vi "Prompt for Step.vi"(8 "error in (no error)":errorcluster, 9 "Index":i32=-1, 11 "Steps":refnum<class "Step.lvclass">[](array[class])) -> (0 "error out":errorcluster, 1 "OK?":bool, 3 "Step":refnum<class "Step.lvclass">)   [LabVIEW 2020, in "MacroAssert.lvlib"]
doc: "Prompts to enter a new step in the profile."
uses:
  MacroAssert.lvlib
  Classes/Step/Step.lvclass
  Classes/Macro/Macro.lvclass
  CTLs/Prompt for Step State Data.ctl
  FaKI State Machine/FaKI State Machine.lvlib
  CTLs/Step Type V3.ctl
panel:
  in  "Save Default":bool
  in  "Step Notes":string
  out "Step Type Description":string
  in  "Repeat":i32 min=0
  in  "Delay":i32=100 min=0
  in  "Step Type":T1
  in  "Cancel":bool
  in  "OK":bool
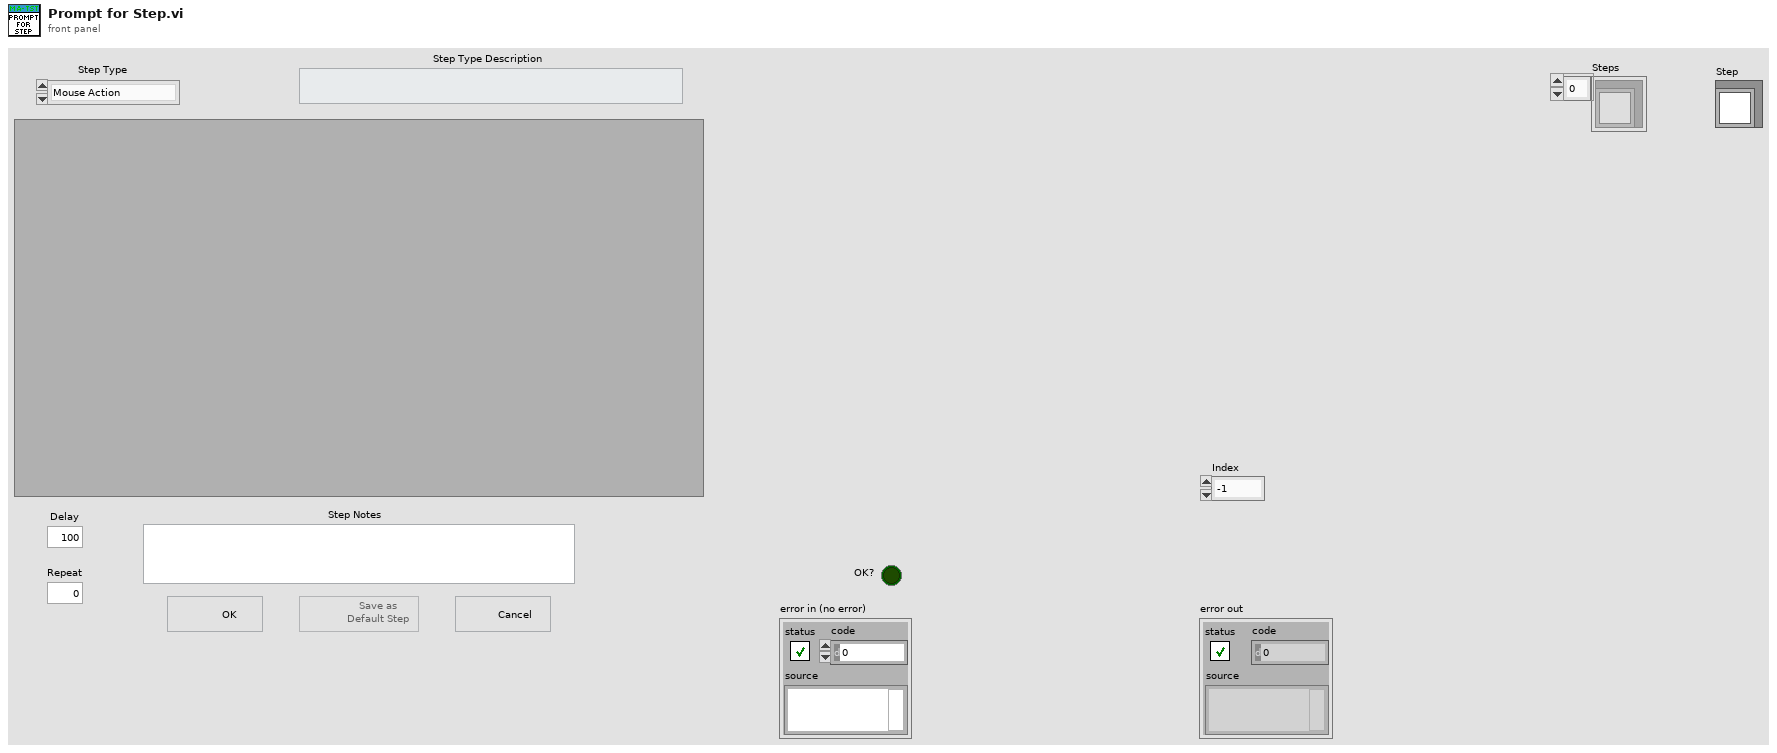
[diagram p1: front panel]
types:
  T1 = typedef "MacroAssert.lvlib/Step Type V3.ctl" = enum16{"Mouse Action", "Keyboard Action", "Window Action", "Timing Action", "Boolean Assertion", "Numeric Assertion", "String Assertion", "Image Assertion"}
  T2 = typedef "MacroAssert.lvlib/Prompt for Step State Data.ctl" = cluster{"Core":cluster{"Current VI Reference":refnum<vi>, "Close Panel on Exit?":bool}, "Mouse Ref":refnum<k1>, "Step":refnum<class "Step.lvclass">, "OK?":bool}
  T3 = enum32{"Invalid", "Standard", "Closed", "Hidden", "Minimized", "Maximized"}
  T4 = enum32{"invalid app kind", "Development System", "Run Time System", "Student Edition", "Embedded LabVIEW", "Evaluation", "Custom"}
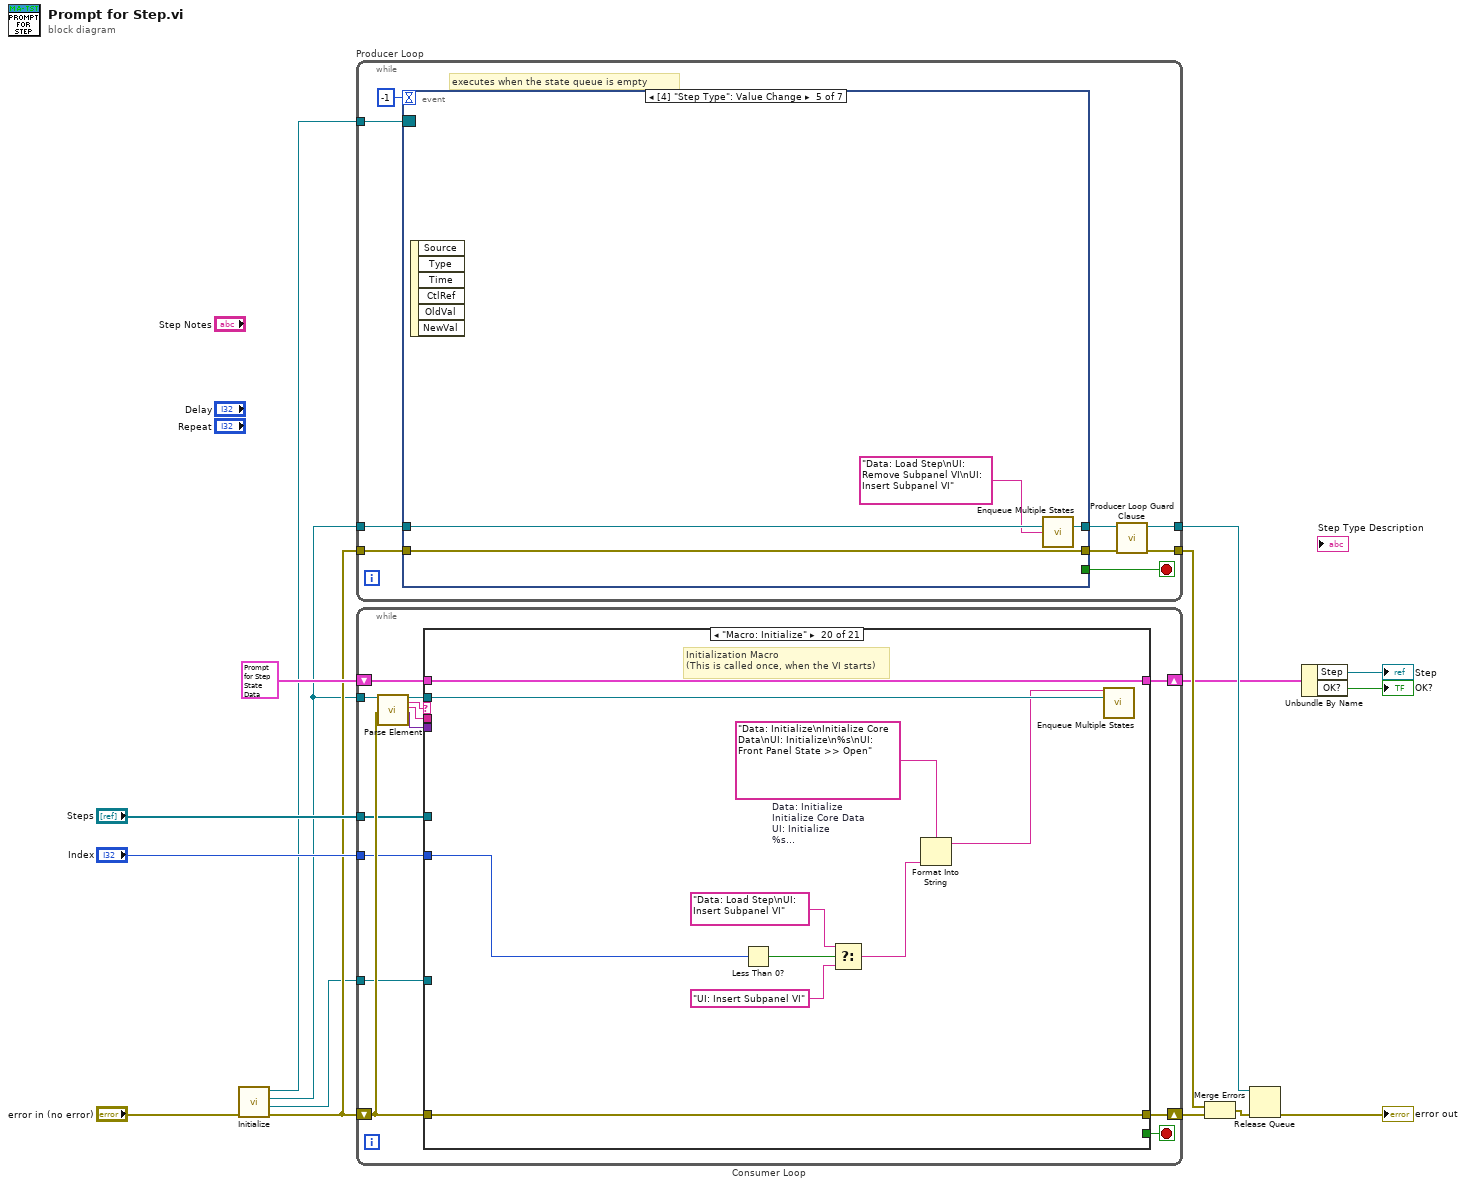
[diagram p0: block diagram]
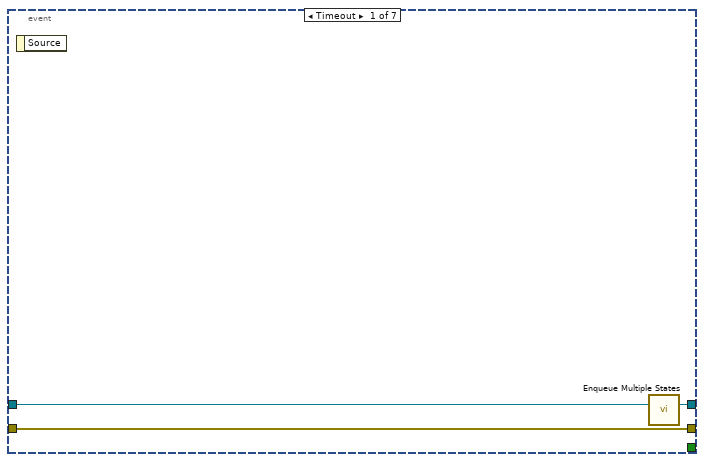
[diagram p2: hidden frame]
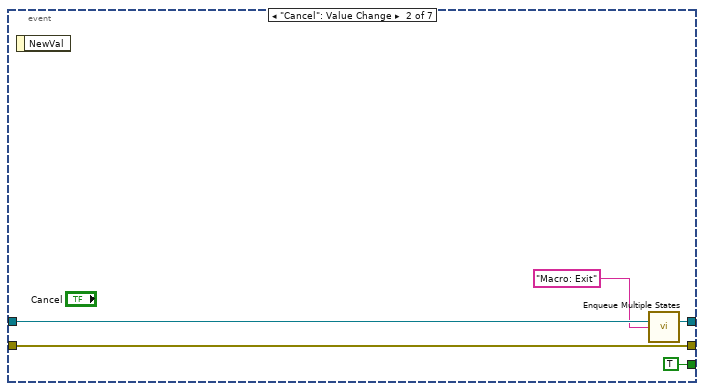
[diagram p3: hidden frame]
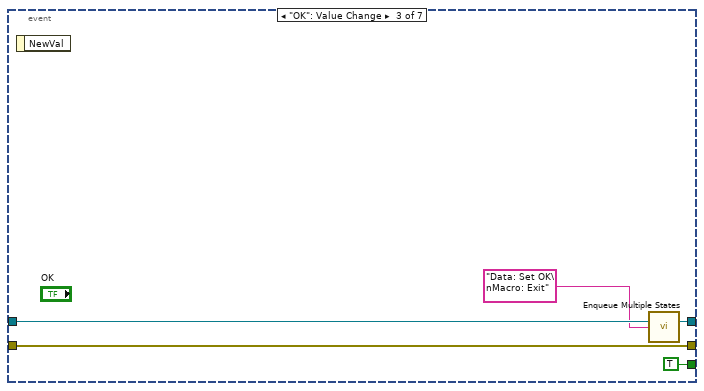
[diagram p4: hidden frame]
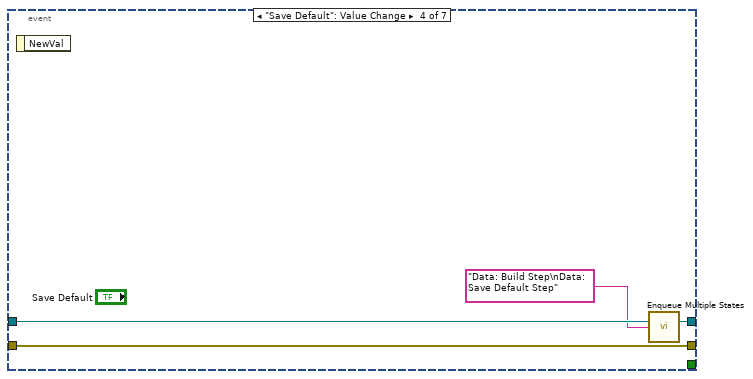
[diagram p5: hidden frame]
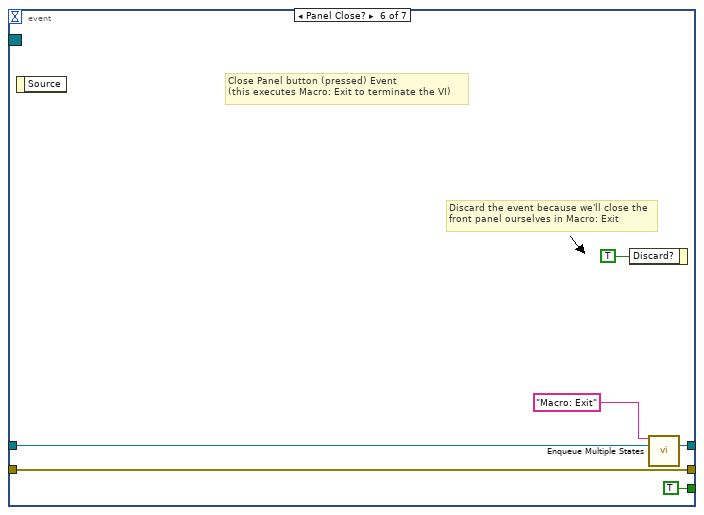
[diagram p6: hidden frame]
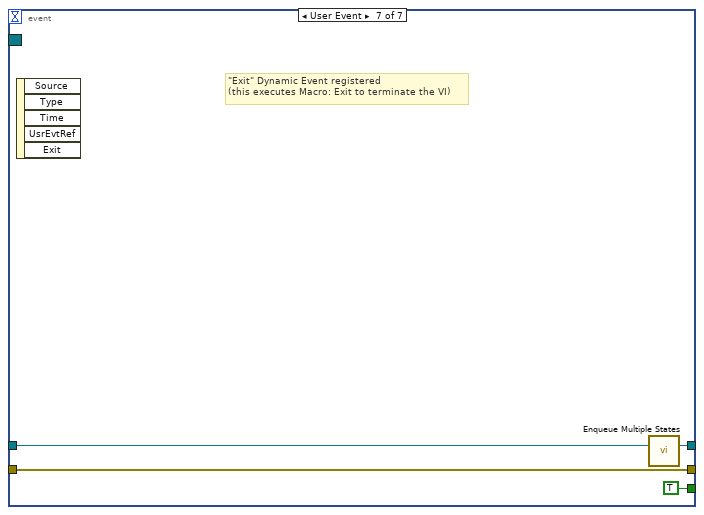
[diagram p7: hidden frame]
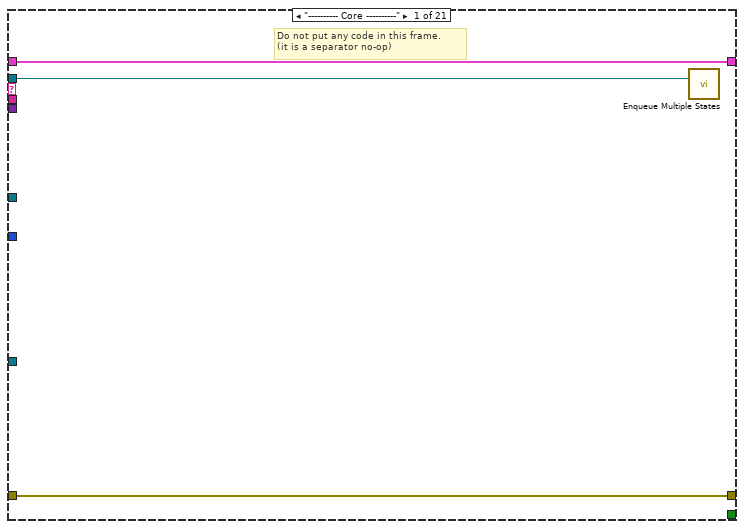
[diagram p8: hidden frame]
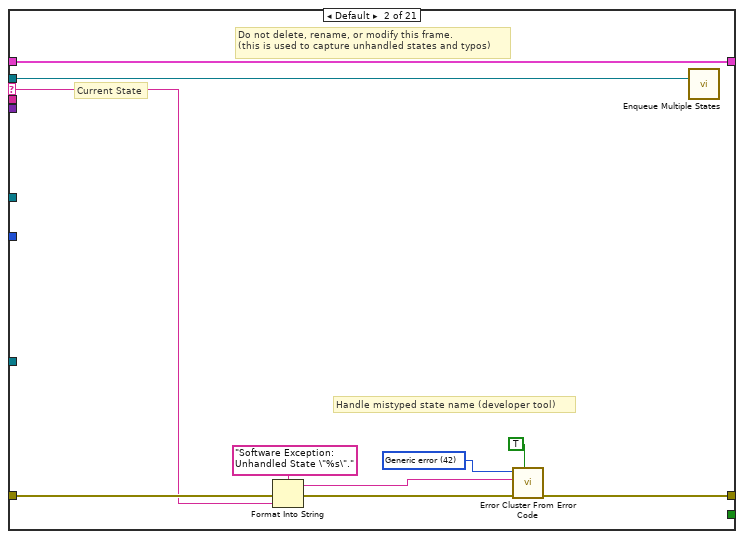
[diagram p9: hidden frame]
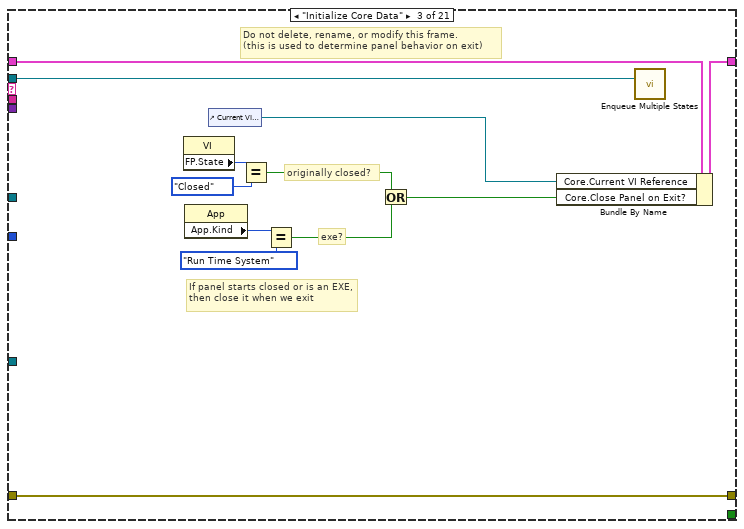
[diagram p10: hidden frame]
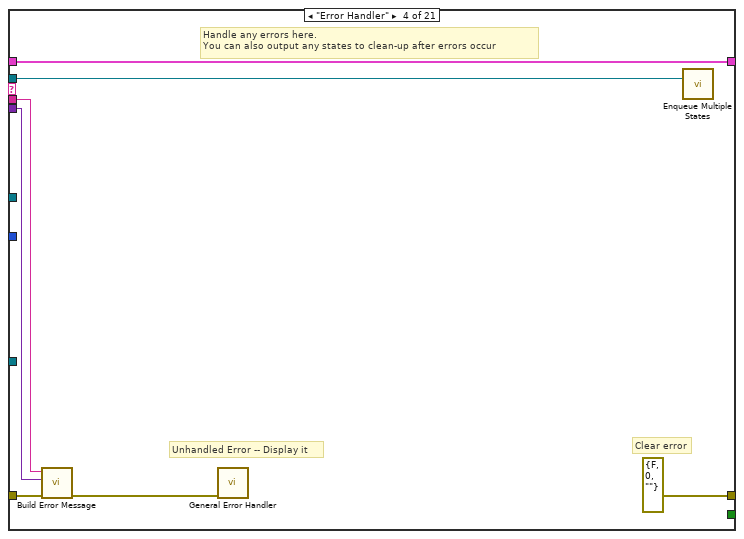
[diagram p11: hidden frame]
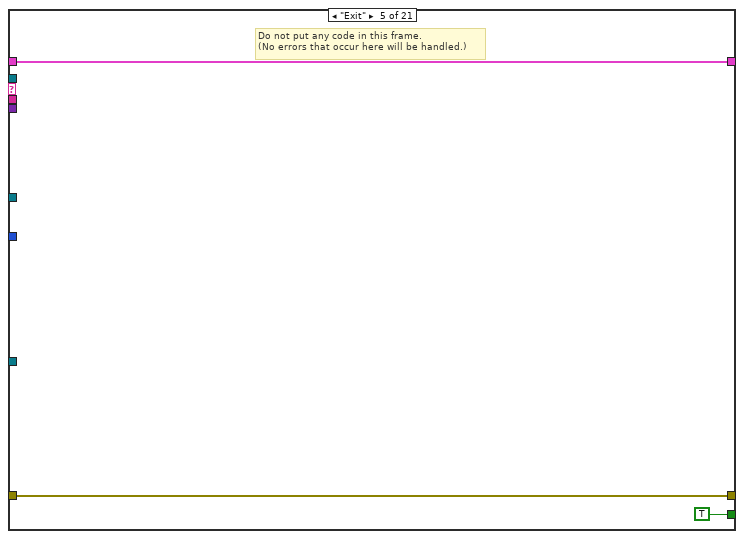
[diagram p12: hidden frame]
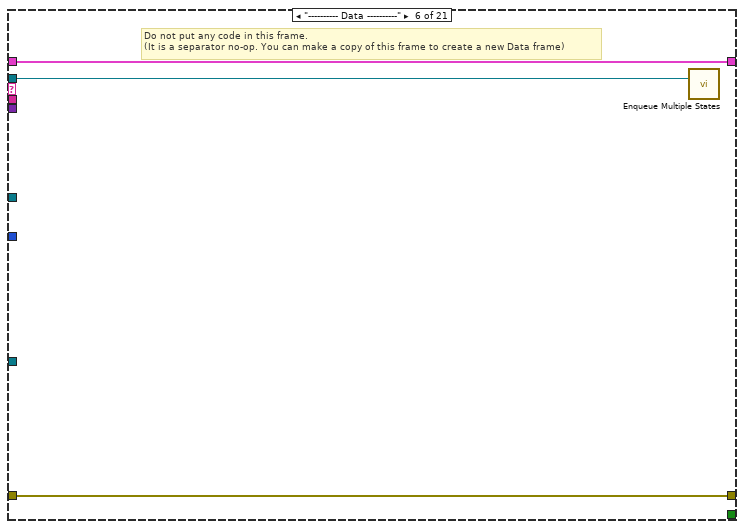
[diagram p13: hidden frame]
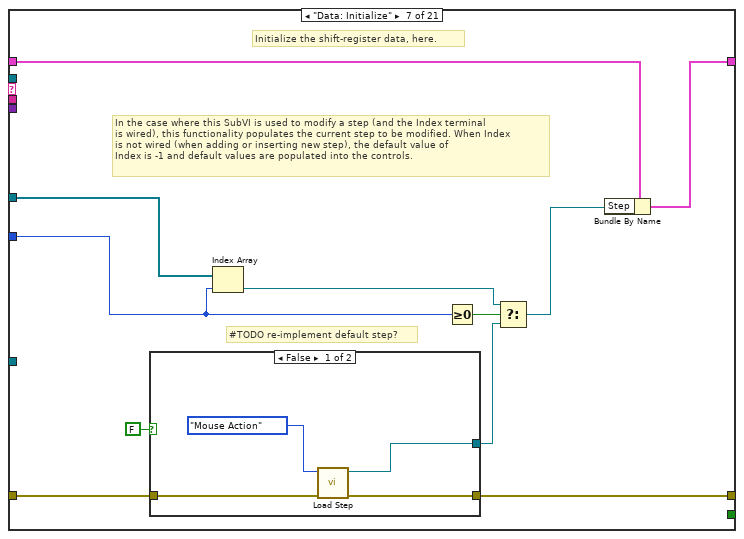
[diagram p14: hidden frame]
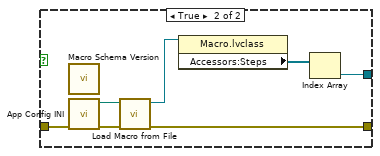
[diagram p15: hidden frame]
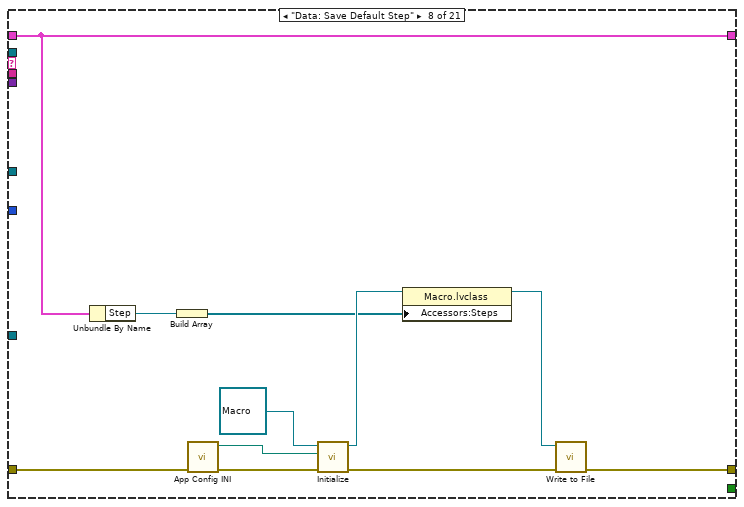
[diagram p16: hidden frame]
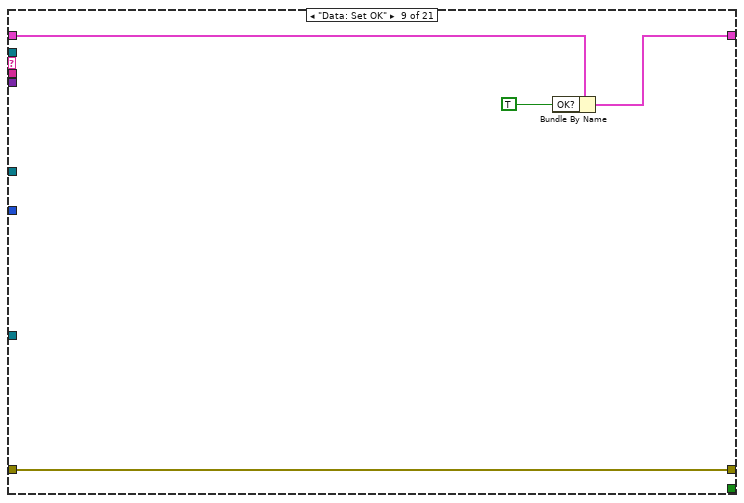
[diagram p17: hidden frame]
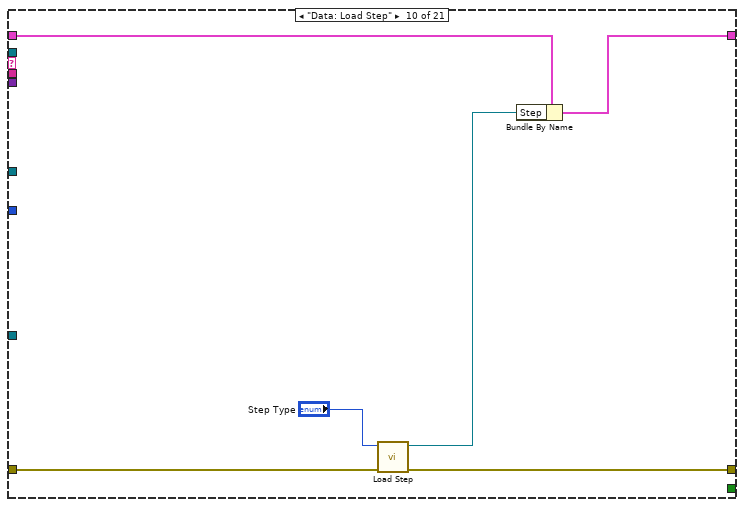
[diagram p18: hidden frame]
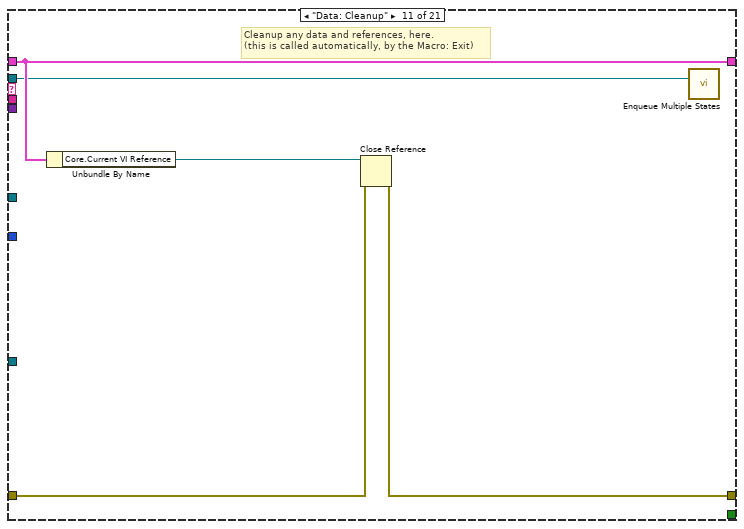
[diagram p19: hidden frame]
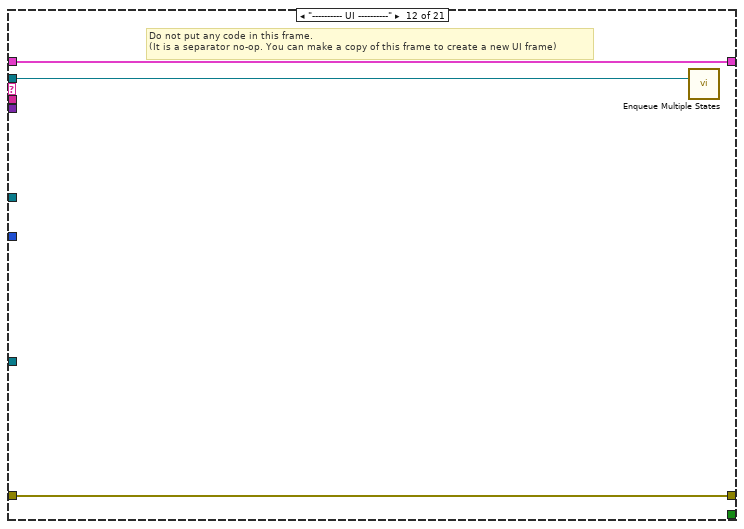
[diagram p20: hidden frame]
diagram:
  n1 = call "Initialize.vi"("error in (no error)"="error in (no error)") -> ("error out"=w6:errorcluster, "Exit Event"=w2:refnum<user-event>, "Queue"=w5:refnum<queue>, "Event Registration Refnum"=w4:refnum<event-registration>)  [unwired: 7 in]
  n2 = while "Producer Loop" {
    tunnel: w4 -> [w17]
    tunnel: w5 -> [w21]
    tunnel: [w18] -> w12
    tunnel: w6 -> [w25]
    tunnel: [w23] -> w15
    stop <- w20 stop-if-true
    # "executes when the state queue is empty"
    n3 = event shown="[4] \"Step Type\": Value Change" {
      selector: w17 -> [_ _ _ _ _ _ _]
      dyn-events: _ -> [_ _ _ _ _ _ _]
      timeout: -1 ("Timeout") -> [_ _ _ _ _ _ _]
      tunnel: [w28 w33 w38 w42 w46 w52 w56] -> w24
      tunnel: w25 -> [w28 w33 w38 w42 w46 w52 w56]
      tunnel: w21 -> [w26 w32 w37 w41 w45 w49 w55]
      tunnel: [w27 w31 w36 w40 w44 w48 w54] -> w19
      tunnel: [_ TRUE TRUE _ _ TRUE TRUE] -> w20
      event Timeout {
        n4 = event-data() -> ()  [unwired: 1 in, 1 out]
        n5 = call "Enqueue Multiple States.vi"("queue in"=w26) -> ("queue out"=w27:refnum<queue>)  [unwired: 14 in]
      }
      event "Cancel": Value Change {
        n6 = event-data() -> ()  [unwired: 1 in, 1 out]
        n7 = call "Enqueue Multiple States.vi"("queue in"=w32, "State(s) at Back"="Macro: Exit") -> ("queue out"=w31:refnum<queue>)  [unwired: 13 in]
      }
      event "OK": Value Change {
        n8 = event-data() -> ()  [unwired: 1 in, 1 out]
        n9 = call "Enqueue Multiple States.vi"("queue in"=w37, "State(s) at Back"="Data: Set OK\nMacro: Exit") -> ("queue out"=w36:refnum<queue>)  [unwired: 13 in]
      }
      event "Save Default": Value Change {
        n10 = event-data() -> ()  [unwired: 1 in, 1 out]
        n11 = call "Enqueue Multiple States.vi"("queue in"=w41, "State(s) at Back"="Data: Build Step\nData: Save Default Step") -> ("queue out"=w40:refnum<queue>)  [unwired: 13 in]
      }
      event Value Change {
        n12 = event-data() -> ()  [unwired: 1 in, 6 out]
        n13 = call "Enqueue Multiple States.vi"("queue in"=w45, "State(s) at Back"="Data: Load Step\nUI: Remove Subpanel VI\nUI: Insert Subpanel VI") -> ("queue out"=w44:refnum<queue>)  [unwired: 13 in]
      }
      event Panel Close? {
        # "Discard the event because we'll close the front panel ourselves in Macro: Exit"
        # "Close Panel button (pressed) Event\n(this executes Macro: Exit to terminate the VI)"
        n14 = event-data() -> ()  [unwired: 1 in, 1 out]
        n15 = event-data("Discard?"=TRUE) -> ()  [unwired: 1 in, 1 out]
        n16 = call "Enqueue Multiple States.vi"("State(s) at Front"="Macro: Exit", "queue in"=w49) -> ("queue out"=w48:refnum<queue>)  [unwired: 13 in]
      }
      event User Event {
        # "\"Exit\" Dynamic Event registered\n(this executes Macro: Exit to terminate the VI)"
        n17 = event-data() -> ()  [unwired: 1 in, 5 out]
        n18 = call "Enqueue Multiple States.vi"("queue in"=w55) -> ("queue out"=w54:refnum<queue>)  [unwired: 14 in]
      }
    }
    n19 = call "Producer Loop Guard Clause.vi"("error in (no error)"=w24, "queue in"=w19) -> ("error out"=w23:errorcluster, "queue out"=w18:refnum<queue>)  [unwired: 8 in]
  }
  n20 = while "Consumer Loop" {
    shift-right: [w66] -> w8
    shift-left: T2 {"Core"={"Current VI Reference"=refnum, "Close Panel on Exit?"=FALSE}, "Mouse Ref"=refnum, "Step"=refnum, "OK?"=FALSE} ("Prompt for Step State Data") -> [w57]
    shift-right: [w69] -> w16
    shift-left: w6 -> [w68]
    tunnel: w5 -> [w65]
    tunnel: w2 -> [w60]
    tunnel: "Steps" -> [w59]
    tunnel: "Index" -> [w58]
    stop <- w67 stop-if-true
    n21 = call "Parse Element.vi"("queue in"=w65, "error in (no error)"=w68) -> ("queue out"=w64:refnum<queue>, "State"=w63:string, "Arg"=w62:string, "Data"=w61:variant)  [unwired: 14 in]
    n22 = case shown="\"Macro: Initialize\"" w63 {
      selector: w63 -> [_ w74 _ _ _ _ _ _ _ _ _ _ _ _ _ _ _ _ _ _ _]
      tunnel: w64 -> [w70 w73 w83 w97 _ w105 _ _ _ _ w152 w156 w161 w164 w165 w174 _ _ w258 w269 w279]
      tunnel: w62 -> [_ _ _ w95 _ _ _ _ _ _ _ _ _ _ w166 w175 _ _ _ _ _]
      tunnel: w57 -> [w71 w76 w89 w98 w103 w106 w117 w139 w144 w150 w153 w157 w160 w163 w167 w177 w246 w257 w259 w268 w283]
      tunnel: [w72 w81 w94 errorcluster {"status"=FALSE, "code"=0, "source"=""} ("error out") w104 w107 w110 w132 w142 w146 w151 w158 w159 w162 w168 w178 w248 w255 w260 w270 w272] -> w69
      tunnel: w68 -> [w72 w80 w94 w100 w104 w107 w118 w140 w142 w147 w155 w158 w159 w162 w169 w179 w247 w256 w260 w270 w273]
      tunnel: [_ _ _ _ TRUE _ _ _ _ _ _ _ _ _ _ _ _ _ _ _ _] -> w67
      tunnel: [w71 w76 w93 w98 w103 w106 w116 w139 w143 w149 w153 w157 w160 w163 w167 w177 w245 w257 w259 w268 w283] -> w66
      tunnel: w61 -> [_ _ _ w96 _ _ _ _ _ _ _ _ _ _ _ _ _ _ _ _ _]
      tunnel: w60 -> [_ _ _ _ _ _ _ _ _ _ _ _ _ _ _ _ _ _ _ _ w274]
      tunnel: w59 -> [_ _ _ _ _ _ w113 _ _ _ _ _ _ _ _ _ _ _ _ _ _]
      tunnel: w58 -> [_ _ _ _ _ _ w112 _ _ _ _ _ _ _ _ _ _ _ _ w267 _]
      frame "---------- Core ----------" {
        # "Do not put any code in this frame.\n(it is a separator no-op)"
        n23 = call "Enqueue Multiple States.vi"("queue in"=w70) -> ()  [unwired: 14 in, 1 out]
      }
      frame Default {
        w78 = 42 items=["No error", "Argument error", "Memory is full", "Out of zone", "End of file", "File already open", "Generic file I/O error", "File not found", "File permission error", "Disk is full", "Duplicate path", "Too many files open", "System feature not enabled", "Resource file not found", "Cannot add resource", "Resource not found", "Image not found", "Image memory error", "Pen does not exist", "Config type invalid", "Config token not found", "Config parse error", "Config memory error", "Bad external code format", "Bad external code offset", "External code not present", "Null window", "Destroy window error", "Null menu", "Print aborted", "Bad print record", "Print driver error", "Windows error during printing", "Memory error during printing", "Print dialog error", "Generic print error", "Invalid device refnum", "Device not found", "Device parameter error", "Device unit error", "Cannot open device", "Device call aborted", "Generic error", "Cancelled by user", "Object ID too low", "Object ID too high", "Object not in heap", "Unknown heap", "Unknown object (invalid DefProc)", "Unknown object (DefProc not in table)", "Message out of range", "Invalid (null) method", "Unknown message", "Manager call not supported", "Bad address", "Network operation in progress", "Network operation timed out", "Connection is busy", "Network attribute not supported", "Network error", "Address in use", "System out of memory", "Connection aborted", "Connection refused", "Not connected", "Already connected", "Connection closed", "Initialization error (interapplication manager)", "Bad occurrence", "Wait on unbound occurrence handler", "Occurrence queue overflow", "Datalog type conflict", "Unused", "Unrecognized type (interapplication manager)", "Memory corrupt", "Failed to make temporary DLL", "Old CIN version", "Drag socket not found", "Failed to load drop-object", "Failed to register OLE object", "Failed to release OLE object", "Format specifier type mismatch", "Unknown format specifier", "Too few format specifiers", "Too many format specifiers", "Scan failed", "Newer CIN version", "Error converting to variant", "Runtime menu error", "Password tampered", "Variant attribute not found", "Incompatible variant data type", "Event data is not available", "Event Store is not present", "Occurrence is not found", "Event Queue is not created", "Event info is not available", "Refnum passed is NULL", "Error retrieving Class GUID", "Error retrieving CoClass GUID", "Error retrieving TypeLib GUID.", "Bad built application magic bytes.", "Specific driver is different from the specific driver associated with the Logical Name.", "There is no session opened to the class driver.", "Max Error", "MAX - Error with config objects", "MAX - Error loading configuration", "MAX - Group not supported"]
        # "Current State"
        # "Do not delete, rename, or modify this frame.\n(this is used to capture unhandled states and typos)"
        # "Handle mistyped state name (developer tool)"
        n24 = Format Into String(format string="Software Exception: Unhandled State \"%s\"." ("message"), error in=w80, w74) -> (resulting string=w77:string, error out=w82:errorcluster)  [unwired: 1 in]
        n25 = call <vilib>:"Error Cluster From Error Code.vi"("show call chain? (False)"=TRUE, "error in (no error)"=w82, "error message (\"\")"=w77, "error code (0)"=w78) -> ("error out"=w81:errorcluster)  [unwired: 5 in]
        n26 = call "Enqueue Multiple States.vi"("queue in"=w73) -> ()  [unwired: 14 in, 1 out]
      }
      frame "Initialize Core Data" {
        # "Do not delete, rename, or modify this frame.\n(this is used to determine panel behavior on exit)"
        # "originally closed?"
        # "exe?"
        # "If panel starts closed or is an EXE, then close it when we exit"
        n27 = property class="VI"() -> ("FP.State"=w86:T3)  [unwired: 2 in, 2 out]
        n28 = property class="App"() -> ("App.Kind"=w92:T4)  [unwired: 2 in, 2 out]
        n29 = control-ref of="Current VI Reference"() -> (w87:refnum<vi>)
        n30 = Equal?(x=w86, y=T3."Closed" ("Front Panel Window:State")) -> (x = y?=w84:bool)
        n31 = Equal?(x=w92, y=T4."Run Time System" ("Application:Kind")) -> (x = y?=w90:bool)
        n32 = Or(x=w84, y=w90) -> (x .or. y?=w88:bool)
        n33 = Bundle By Name(cluster=w89, "Core.Current VI Reference"=w87, "Core.Close Panel on Exit?"=w88) -> (w93:T2)
        n34 = call "Enqueue Multiple States.vi"("queue in"=w83) -> ()  [unwired: 14 in, 1 out]
      }
      frame "Error Handler" {
        # "Unhandled Error -- Display it"
        # "Handle any errors here.\nYou can also output any states to clean-up after errors occur"
        # "Clear error"
        n35 = call "Build Error Message.vi"("error in (no error)"=w100, "Data"=w96, "Arg"=w95) -> ("error out"=w99:errorcluster)  [unwired: 8 in]
        n36 = call <vilib>:"General Error Handler.vi"("error in (no error)"=w99) -> ()  [unwired: 10 in, 5 out]
        n37 = call "Enqueue Multiple States.vi"("queue in"=w97) -> ()  [unwired: 14 in, 1 out]
      }
      frame "Exit" {
        # "Do not put any code in this frame.\n(No errors that occur here will be handled.)"
      }
      frame "---------- Data ----------" {
        # "Do not put any code in this frame.\n(It is a separator no-op. You can make a copy of this frame to create a new Data frame)"
        n38 = call "Enqueue Multiple States.vi"("queue in"=w105) -> ()  [unwired: 14 in, 1 out]
      }
      frame "Data: Initialize" {
        # "#TODO re-implement default step?"
        # "In the case where this SubVI is used to modify a step (and the Index terminal\nis wired), this functionality populates the current step to be modified. When Index\nis not wired (when adding or inserting new step), the default value of\nIndex is -1 and default values are populated into the controls."
        # "Initialize the shift-register data, here."
        n39 = case shown="False" FALSE {
          tunnel: w118 -> [w122 w129]
          tunnel: [w121 w126] -> w110
          tunnel: [w120 w125] -> w109
          frame False {
            n40 = call "Load Step.vi"("error in (no error)"=w122, "Step Type"=Step_Type_V3."Mouse Action") -> ("error out"=w121:errorcluster, "Step"=w120:refnum<class "Step.lvclass">)  [unwired: 8 in]
          }
          frame True {
            n41 = call "Macro Schema Version.vi"() -> ()  [unwired: 10 in, 2 out]
            n42 = call "App Config INI.vi"("error in (no error)"=w129) -> ("error out"=w128:errorcluster, "App Config"=w127:path)  [unwired: 9 in]
            n43 = call "Load Macro from File.vi"("error in (no error)"=w128, "Path"=w127) -> ("error out"=w126:errorcluster, "Macro"=w124:refnum<class "Macro.lvclass">)  [unwired: 8 in]
            n44 = property class="Macro.lvclass"(reference=w124) -> ("Accessors:Steps"=w123:refnum<class "Step.lvclass">[])  [unwired: 1 in, 2 out]
            n45 = Index Array(array=w123) -> (element=w125:refnum<class "Step.lvclass">)  [unwired: 1 in]
          }
        }
        n46 = Index Array(array=w113, index=w112) -> (element=w115:refnum<class "Step.lvclass">)
        n47 = Greater Or Equal To 0?(x=w112) -> (x >= 0?=w114:bool)
        n48 = Select(t=w115, s=w114, f=w109) -> (s? t:f=w111:refnum<class "Step.lvclass">)
        n49 = Bundle By Name(cluster=w117, "Step"=w111) -> (w116:T2)
      }
      frame "Data: Save Default Step" {
        n50 = Unbundle By Name(w139) -> ("Step"=w138:refnum<class "Step.lvclass">)
        n51 = Build Array(w138) -> (w130:refnum<class "Step.lvclass">[])
        n52 = call "App Config INI.vi"("error in (no error)"=w140) -> ("error out"=w137:errorcluster, "App Config"=w136:path)  [unwired: 9 in]
        n53 = call-dynamic "Initialize.vi"("error in (no error)"=w137, "Path"=w136, "Macro in"=refnum<class "Macro.lvclass"> refnum) -> ("error out"=w134:errorcluster, "Macro out"=w133:refnum<class "Macro.lvclass">)  [unwired: 7 in]
        n54 = property class="Macro.lvclass"(reference=w133, "Accessors:Steps"=w130) -> (reference out=w131:refnum<class "Macro.lvclass">)  [unwired: 1 in, 1 out]
        n55 = call-dynamic "Write to File.vi"("error in (no error)"=w134, "Macro in"=w131) -> ("error out"=w132:errorcluster)  [unwired: 8 in, 1 out]
      }
      frame "Data: Set OK" {
        n56 = Bundle By Name(cluster=w144, "OK?"=TRUE) -> (w143:T2)
      }
      frame "Data: Load Step" {
        n57 = call "Load Step.vi"("error in (no error)"=w147, "Step Type"="Step Type") -> ("error out"=w146:errorcluster, "Step"=w145:refnum<class "Step.lvclass">)  [unwired: 8 in]
        n58 = Bundle By Name(cluster=w150, "Step"=w145) -> (w149:T2)
      }
      frame "Data: Cleanup" {
        # "Cleanup any data and references, here.\n(this is called automatically, by the Macro: Exit)"
        n59 = Unbundle By Name(w153) -> ("Core.Current VI Reference"=w154:refnum<vi>)
        n60 = Close Reference(reference=w154, error in (no error)=w155) -> (error out=w151:errorcluster)
        n61 = call "Enqueue Multiple States.vi"("queue in"=w152) -> ()  [unwired: 14 in, 1 out]
      }
      frame "---------- UI ----------" {
        # "Do not put any code in this frame.\n(It is a separator no-op. You can make a copy of this frame to create a new UI frame)"
        n62 = call "Enqueue Multiple States.vi"("queue in"=w156) -> ()  [unwired: 14 in, 1 out]
      }
      frame "UI: Initialize" {
        # "Initialize the User Interface, here.\n(this is called automatically, by the Macro: Init)"
        n63 = call "Enqueue Multiple States.vi"("queue in"=w161) -> ()  [unwired: 14 in, 1 out]
      }
      frame "UI: Uninitialize" {
        # "Uninitialize the User Interface, here.\n(this is called automatically, by the Macro: Exit)"
        n64 = call "Enqueue Multiple States.vi"("queue in"=w164) -> ()  [unwired: 14 in, 1 out]
      }
      frame "UI: Cursor Set" {
        # "Argument"
        # "Set and Unset Cursor Busy.\n(Usage: \"UI: Cursor Set >> Busy|Idle\")"
        n65 = case shown="\"Idle\", Default" w166 {
          tunnel: w169 -> [w171 w173]
          tunnel: [w170 w172] -> w168
          frame "Idle", Default {
            n66 = call <vilib>:"Unset Busy.vi"("error in (no error)"=w171) -> ("error out"=w170:errorcluster)  [unwired: 10 in]
          }
          frame "Busy" {
            n67 = call <vilib>:"Set Busy.vi"("error in (no error)"=w173) -> ("error out"=w172:errorcluster)  [unwired: 9 in, 1 out]
          }
        }
        n68 = call "Enqueue Multiple States.vi"("queue in"=w165) -> ()  [unwired: 14 in, 1 out]
      }
      frame "UI: Front Panel State" {
        # "Argument"
        # "Set Front Panel Open or Closed\n(Usage: \"UI: Front Panel State >> Open|Close\")"
        n69 = Unbundle By Name(w177) -> ("Core.Current VI Reference"=w176:refnum<vi>)
        n70 = case shown="\"Open\", \"Standard\", Default" w175 {
          tunnel: w179 -> [w186 w200 w212 w225 w238]
          tunnel: [w187 w201 w213 w226 w239] -> w178
          tunnel: w176 -> [w184 w198 w210 w223 w236]
          frame "Open", "Standard", Default {
            w180 = T3."Standard" ("State")
            n71 = property class="VI"(reference=w184, error in=w186) -> (reference out=w183:refnum<vi>, error out=w185:errorcluster, "FP.State"=w182:T3)
            n72 = Not Equal?(x=w182, y=w180) -> (x != y?=w181:bool)
            n73 = case shown="True" w181 {
              tunnel: [w192 w193] -> w187
              tunnel: w185 -> [w191 w193]
              tunnel: w183 -> [w189 _]
              tunnel: w180 -> [w188 _]
              frame True {
                n74 = invoke class="VI" method="FP.Open"(reference=w189, error in=w191, "Activate"=TRUE, "State"=w188) -> (error out=w192:errorcluster)  [unwired: 1 in, 4 out]
              }
              frame False {
              }
            }
          }
          frame "Close", "Closed" {
            n75 = property class="VI"(reference=w198, error in=w200) -> (reference out=w197:refnum<vi>, error out=w199:errorcluster, "FP.State"=w195:T3)
            n76 = Not Equal?(x=w195, y=T3."Closed" ("Front Panel Window:State")) -> (x != y?=w194:bool)
            n77 = case shown="True" w194 {
              tunnel: [w202 w205] -> w201
              tunnel: w199 -> [w202 w204]
              tunnel: w197 -> [_ w203]
              frame False {
              }
              frame True {
                n78 = invoke class="VI" method="FP.Close"(reference=w203, error in=w204) -> (error out=w205:errorcluster)  [unwired: 1 in, 2 out]
              }
            }
          }
          frame "Hidden", "Hide" {
            w206 = T3."Hidden" ("State")
            n79 = property class="VI"(reference=w210, error in=w212) -> (reference out=w209:refnum<vi>, error out=w211:errorcluster, "FP.State"=w208:T3)
            n80 = Not Equal?(x=w208, y=w206) -> (x != y?=w207:bool)
            n81 = case shown="True" w207 {
              tunnel: [w217 w218] -> w213
              tunnel: w211 -> [w216 w218]
              tunnel: w209 -> [w215 _]
              tunnel: w206 -> [w214 _]
              frame True {
                n82 = invoke class="VI" method="FP.Open"(reference=w215, error in=w216, "State"=w214) -> (error out=w217:errorcluster)  [unwired: 2 in, 4 out]
              }
              frame False {
              }
            }
          }
          frame "Minimize", "Minimized" {
            w219 = T3."Minimized" ("State")
            n83 = property class="VI"(reference=w223, error in=w225) -> (reference out=w222:refnum<vi>, error out=w224:errorcluster, "FP.State"=w221:T3)
            n84 = Not Equal?(x=w221, y=w219) -> (x != y?=w220:bool)
            n85 = case shown="True" w220 {
              tunnel: [w230 w231] -> w226
              tunnel: w224 -> [w229 w231]
              tunnel: w222 -> [w228 _]
              tunnel: w219 -> [w227 _]
              frame True {
                n86 = invoke class="VI" method="FP.Open"(reference=w228, error in=w229, "State"=w227) -> (error out=w230:errorcluster)  [unwired: 2 in, 4 out]
              }
              frame False {
              }
            }
          }
          frame "Maximize", "Maximized" {
            w232 = T3."Maximized" ("State")
            n87 = property class="VI"(reference=w236, error in=w238) -> (reference out=w235:refnum<vi>, error out=w237:errorcluster, "FP.State"=w234:T3)
            n88 = Not Equal?(x=w234, y=w232) -> (x != y?=w233:bool)
            n89 = case shown="True" w233 {
              tunnel: [w243 w244] -> w239
              tunnel: w237 -> [w242 w244]
              tunnel: w235 -> [w241 _]
              tunnel: w232 -> [w240 _]
              frame True {
                n90 = invoke class="VI" method="FP.Open"(reference=w241, error in=w242, "State"=w240) -> (error out=w243:errorcluster)  [unwired: 2 in, 4 out]
              }
              frame False {
              }
            }
          }
        }
        n91 = call "Enqueue Multiple States.vi"("queue in"=w174) -> ()  [unwired: 14 in, 1 out]
      }
      frame "UI: Insert Subpanel VI" {
        n92 = in-place {
          in-place-border: [w253] -> w248
          in-place-border: w247 -> [w251]
          n93 = in-place-cluster #1(w246) -> ("Step"=w250:refnum<class "Step.lvclass">)
          n94 = control-ref of="Sub Panel"() -> (w252:refnum<vi>)
          n95 = call-dynamic "Prompt for Step.vi"("error in (no error)"=w251, "Subpanel Ref"=w252, "Step in"=w250) -> ("error out"=w253:errorcluster, "Step out"=w249:refnum<class "Step.lvclass">)  [unwired: 7 in]
          n96 = in-place-cluster #1("Step"=w249) -> (w245:T2)
        }
      }
      frame "UI: Remove Subpanel VI" {
        n97 = control-ref of="Sub Panel"() -> (w254:refnum<vi>)
        n98 = invoke class="SubPnl" method="Remove VI"(reference=w254, error in=w256) -> (error out=w255:errorcluster)  [unwired: 1 in, 2 out]
      }
      frame "---------- Macro ----------" {
        # "Do not put any code in this frame.\n(It is a separator no-op. You can make a copy of this frame to create a new Macro frame)"
        n99 = call "Enqueue Multiple States.vi"("queue in"=w258) -> ()  [unwired: 14 in, 1 out]
      }
      frame "Macro: Initialize" {
        w265 = "Data: Initialize\nInitialize Core Data\nUI: Initialize\n%s\nUI: Front Panel State >> Open"  # Data: Initialize Initialize Core Data UI: Initialize %s UI: Front Panel State >> Open
        # "Initialization Macro\n(This is called once, when the VI starts)"
        n100 = Less Than 0?(x=w267) -> (x < 0?=w266:bool)
        n101 = Select(t="Data: Load Step\nUI: Insert Subpanel VI", s=w266, f="UI: Insert Subpanel VI") -> (s? t:f=w262:string)
        n102 = Format Into String(format string=w265, w262) -> (resulting string=w261:string)  [unwired: 2 in, 1 out]
        n103 = call "Enqueue Multiple States.vi"("State(s) at Front"=w261, "queue in"=w269) -> ()  [unwired: 13 in, 1 out]
      }
      frame "Macro: Exit" {
        # "Exit Macro\n(This is called once, when the VI exits)"
        n104 = Unbundle By Name(w283) -> ("Core.Close Panel on Exit?"=w282:bool)
        n105 = Generate User Event(user event=w274, event data cluster=FALSE ("event data"), error in=w273) -> (error out=w272:errorcluster)  [unwired: 1 in, 1 out]
        n106 = Select(t="UI: Front Panel State >> Close\n", s=w282, f="") -> (s? t:f=w278:string)
        n107 = Concatenate Strings("UI: Uninitialize\n", w278, "Data: Cleanup\nExit") -> (w276:string)
        n108 = call "Enqueue Multiple States.vi"("State(s) at Front"=w276, "queue in"=w279) -> ()  [unwired: 13 in, 1 out]
      }
    }
  }
  n109 = Merge Errors(w15, w16) -> (w14:errorcluster)
  n110 = Release Queue(queue=w12, error in (no error)=w14) -> (error out=→"error out":errorcluster)  [unwired: 1 in, 2 out]
  n111 = Unbundle By Name(w8) -> ("Step"=→"Step":refnum<class "Step.lvclass">, "OK?"=→"OK?":bool)
